vi "SLL Generate or Inject Custom Error.vi"(6 "No of Callers to add":i32=1, 7 "Case Name":string, 8 "error in":errorcluster, 9 "Description":string, 10 "Error Code":i32, 11 "Error? (T)":bool=TRUE) -> (0 "error out":errorcluster)   [LabVIEW 2013]
doc: "Creates the error cluster given the error status and code.It also adds the specified no of caller vi names and the message to the source.\n\n<B>Note : </B> Custom Error code & error description should be added in the Error code file and it should be attached during building Application (EXE)\n\nThis VI also injects error if this VI is called in the specified sub VI in the error simulation module. This is used to simulate the error in any sub VI of the project and test it. The error can be injected at any sub VI by calling this Vi in that sub VI. The most often used places are driver Vis, where ever there is a user defined error generated.\n\n\n\nCopyright © 2006, Soliton Technologies. All rights reserved."
uses:
  SLL Error Simulation Global.vi
panel:
  # "Inputs"
  # "Outputs"
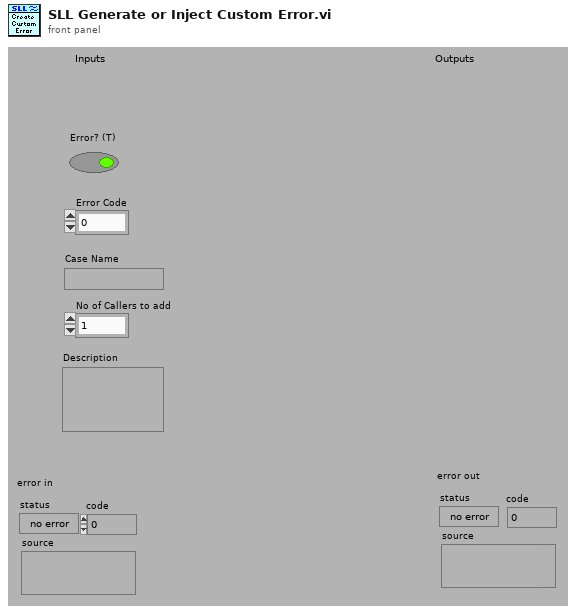
[diagram p1: front panel]
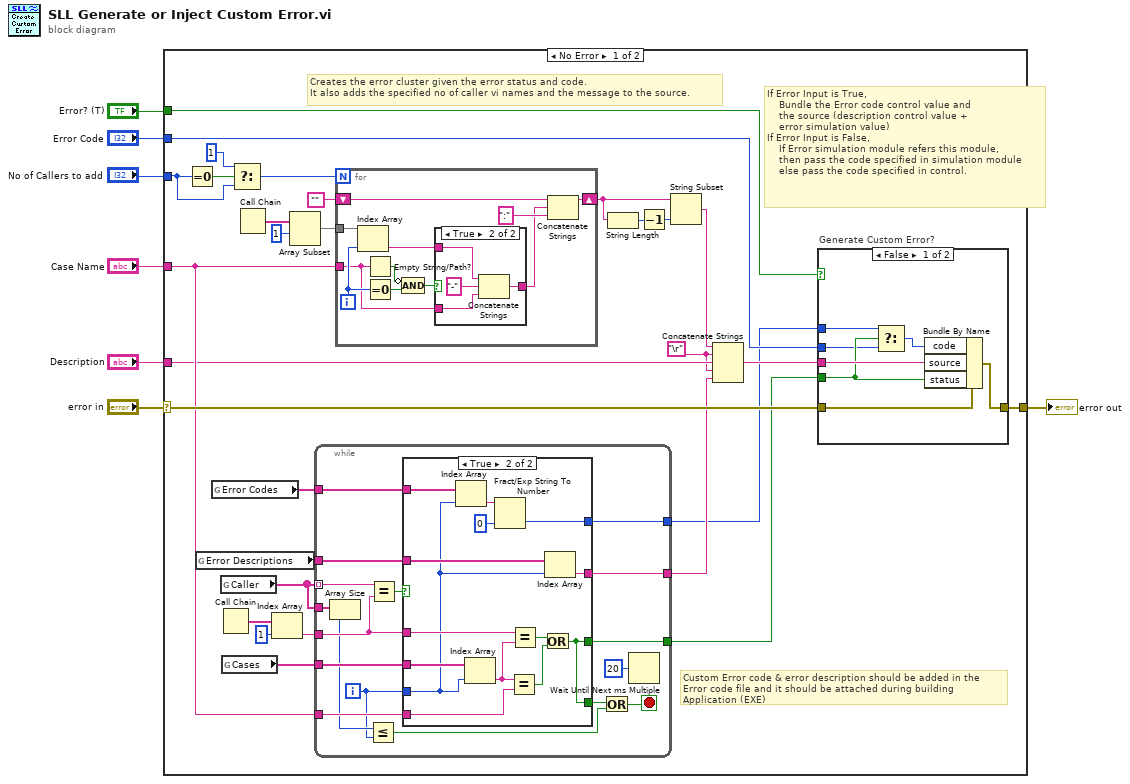
[diagram p0: block diagram]
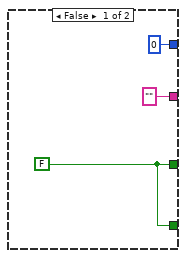
[diagram p2: hidden frame]
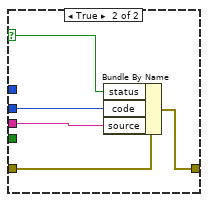
[diagram p3: hidden frame]
diagram:
  n1 = case shown="No Error" "error in" {
    selector: "error in" -> [w36 w100]
    tunnel: [w37 w100] -> w7
    tunnel: "Error? (T)" -> [w18 _]
    tunnel: "No of Callers to add" -> [w34 _]
    tunnel: "Error Code" -> [w35 _]
    tunnel: "Case Name" -> [w19 _]
    tunnel: "Description" -> [w16 _]
    frame No Error {
      w12 = "\r"
      # "If Error Input is True,\n    Bundle the Error code control value and\n    the source (description control value +\n    error simulation value)\nIf Error Input is False,\n    If Error simulation module refers this module,\n    then pass the code specified in simulation module\n    else pass the code specified in control."
      # "Custom Error code & error description should be added in the Error code file and it should be attached during building Application (EXE)"
      # "Creates the error cluster given the error status and code.\nIt also adds the specified no of caller vi names and the message to the source."
      n2 = Equal To 0?(x=w34) -> (x = 0?=w29:bool)
      n3 = global read "SLL Error Simulation Global.vi" "Error Descriptions"() -> (w10:string[])
      n4 = global read "SLL Error Simulation Global.vi" "Error Codes"() -> (w9:string[])
      n5 = global read "SLL Error Simulation Global.vi" "Caller"() -> (w13:string[])
      n6 = Call Chain() -> (call chain=w23:string[])
      n7 = global read "SLL Error Simulation Global.vi" "Cases"() -> (w20:string[])
      n8 = Select(t=1 ("Array Index"), s=w29, f=w34) -> (s? t:f=w27:i32)
      n9 = Call Chain() -> (call chain=w33:string[])
      n10 = Index Array(array=w23, index=1) -> (element=w21:string)
      n11 = Array Subset(array=w33, index=1 ("Array Index")) -> (w31:string[])  [unwired: 1 in]
      n12 = while {
        tunnel: w13 -> [w54] mode=indexing
        tunnel: w21 -> [w50]
        tunnel: w20 -> [w52]
        tunnel: w19 -> [w51]
        tunnel: [w49] -> w14
        tunnel: w13 -> [w45]
        tunnel: [w41] -> w11
        tunnel: w10 -> [w40]
        tunnel: w9 -> [w39]
        tunnel: [w38] -> w8
        i -> [w43]
        stop <- w46 stop-if-true
        n13 = Array Size(array=w45) -> (size(s)=w44:i32)
        n14 = Less Or Equal?(x=w44, y=w43) -> (x <= y?=w42:bool)
        n15 = Equal?(x=w54, y=w50) -> (x = y?=w53:bool)
        n16 = case shown="True" w53 {
          tunnel: w52 -> [_ w71]
          tunnel: w43 -> [_ w59]
          tunnel: w51 -> [_ w70]
          tunnel: w50 -> [_ w69]
          tunnel: [w57 w65] -> w49
          tunnel: [w57 w65] -> w47
          tunnel: ["" ("VI") w64] -> w41
          tunnel: w40 -> [_ w63]
          tunnel: w39 -> [_ w61]
          tunnel: [0 w58] -> w38
          frame False {
            w57 = FALSE
          }
          frame True {
            n17 = Index Array(array=w61, index=w59) -> (element=w60:string)
            n18 = Index Array(array=w71, index=w59) -> (element=w68:string)
            n19 = Fract/Exp String To Number(string=w60, default (0 dbl)=0 ("Error Code")) -> (number=w58:i32)  [unwired: 2 in, 1 out]
            n20 = Equal?(x=w68, y=w70) -> (x = y?=w66:bool)
            n21 = Equal?(x=w69, y=w68) -> (x = y?=w67:bool)
            n22 = Or(x=w67, y=w66) -> (x .or. y?=w65:bool)
            n23 = Index Array(array=w63, index=w59) -> (element=w64:string)
          }
        }
        n24 = Or(x=w47, y=w42) -> (x .or. y?=w46:bool)
        n25 = Wait Until Next ms Multiple(millisecond multiple=u32 20) -> ()  [unwired: 1 out]
      }
      n26 = for {
        N: w27 -> [_]
        tunnel: w31 -> [w94]
        shift-right: [w91] -> w26
        shift-left: "" -> [w92]
        tunnel: w19 -> [w86]
        i -> [w90]
        n27 = Index Array(array=w94, index=w90) -> (element=w84:string)
        n28 = Empty String/Path?(string/path=w86) -> (empty?=w88:bool)
        n29 = Equal To 0?(x=w90) -> (x = 0?=w89:bool)
        n30 = Compound Arithmetic op=AND(invert w88, w89) -> (w87:bool)
        n31 = case shown="True" w87 {
          tunnel: w86 -> [_ w98]
          tunnel: w84 -> [w95 w99]
          tunnel: [w95 w96] -> w85
          frame False {
          }
          frame True {
            n32 = Concatenate Strings(w99, "-" ("string"), w98) -> (w96:string)
          }
        }
        n33 = Concatenate Strings(w92, w85, ":") -> (w91:string)
      }
      n34 = String Length(string=w26) -> (length=w25:i32)
      n35 = Decrement(x=w25) -> (x-1=w24:i32)
      n36 = String Subset(string=w26, length (rest)=w24) -> (substring=w17:string)  [unwired: 1 in]
      n37 = Concatenate Strings(w17, w12, w16, w12, w11) -> (w15:string)
      n38 = case "Generate Custom Error?" shown="False" w18 {
        selector: w18 -> [_ w81]
        tunnel: [w77 w79] -> w37
        tunnel: w36 -> [w78 w83]
        tunnel: w35 -> [w73 w80]
        tunnel: w15 -> [w76 w82]
        tunnel: w14 -> [w75 _]
        tunnel: w8 -> [w74 _]
        frame False {
          n39 = Select(t=w74, s=w75, f=w73) -> (s? t:f=w72:i32)
          n40 = Bundle By Name(cluster=w78, "code"=w72, "source"=w76, "status"=w75) -> (w77:errorcluster)
        }
        frame True {
          n41 = Bundle By Name(cluster=w83, "status"=w81, "code"=w80, "source"=w82) -> (w79:errorcluster)
        }
      }
    }
    frame Error {
      # "Passes the error if there is error in input stage."
    }
  }
  "error out" <- w7
